vi "Remove Error.vi"(8 "error in (no error)":errorcluster, 11 "VISA resource name":refnum<visa-resource-name>) -> (0 "error out":errorcluster, 3 "VISA resource name out":refnum<visa-resource-name>)   [LabVIEW 2013, in "California Instruments iX Series.lvlib"]
doc: "Removes unwanted or known error.\n\n<b>Error(s) Removed:</b>\n1: (1073676294)The number of bytes transferred is equal to the requested input count."
uses:
  California Instruments iX Series.lvlib
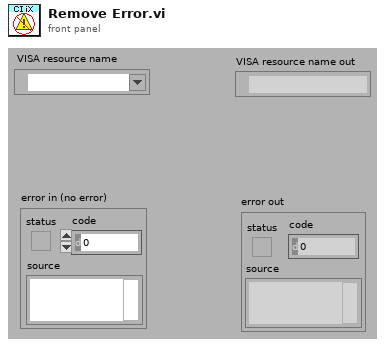
[diagram p1: front panel]
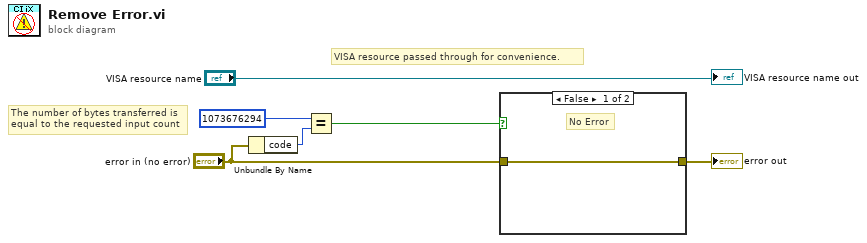
[diagram p0: block diagram]
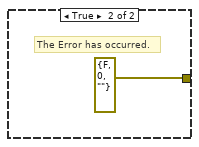
[diagram p2: hidden frame]
diagram:
  # "The number of bytes transferred is equal to the requested input count"
  # "VISA resource passed through for convenience."
  n1 = Unbundle By Name("error in (no error)") -> ("code"=w3:i32)
  n2 = Equal?(x=1073676294, y=w3) -> (x = y?=w1:bool)
  n3 = case shown="False" w1 {
    tunnel: "error in (no error)" -> [w7 _]
    tunnel: [w7 errorcluster {"status"=FALSE, "code"=0, "source"=""} ("error in (no error)")] -> w4
    frame False {
      # "No Error"
    }
    frame True {
      # "The Error has occurred."
    }
  }
  "error out" <- w4
  "VISA resource name out" <- "VISA resource name"
